vi "Fields filled check.vi"(5 "Module stack name (no hyphens; include 320)":string, 6 "Toplayer ID":string, 7 "Baselayer ID":string) -> (0 "Fields fully (not)filled":bool, 1 "Module stack name (no hyphens; include 320) out":string, 2 "Toplayer ID out":string, 3 "Baselayer ID  out":string)   [LabVIEW 2022 SP3, in "Stack.lvclass"]
uses:
  Stack.lvclass
  <vilib>/Utility/error.llb/Trim Whitespace One-Sided.vi
panel:
  out "All not empty":bool
  out "Both not empty":bool
  out "module not empty":bool
  out "module empty":bool
  out "Both empty":bool
  out "All empty":bool
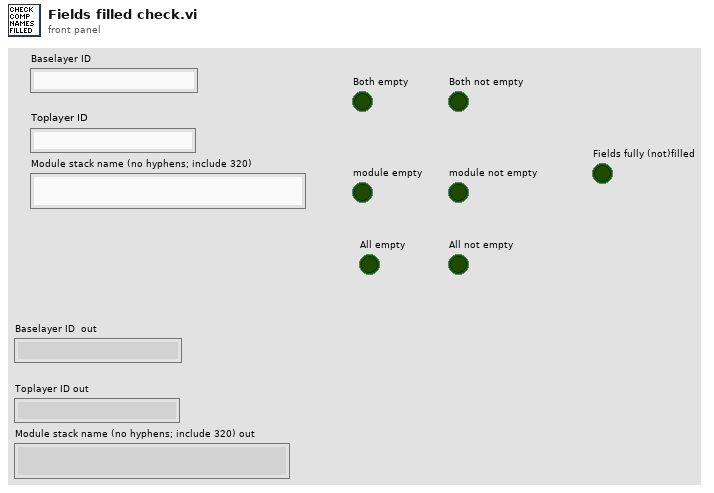
[diagram p1: front panel]
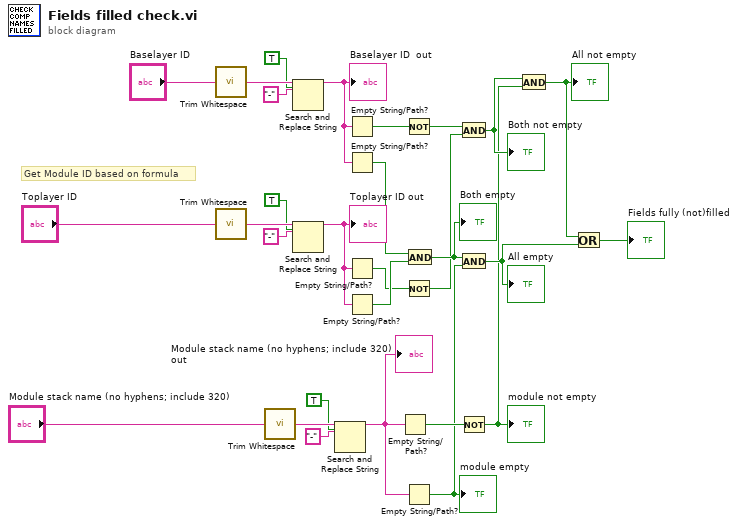
[diagram p0: block diagram]
diagram:
  # "Get Module ID based on formula"
  n1 = call <vilib>:"Trim Whitespace.vi"("string"="Baselayer ID") -> ("trimmed string"=w25:string)  [unwired: 1 in]
  n2 = call <vilib>:"Trim Whitespace.vi"("string"="Toplayer ID") -> ("trimmed string"=w24:string)  [unwired: 1 in]
  n3 = call <vilib>:"Trim Whitespace.vi"("string"="Module stack name (no hyphens; include 320)") -> ("trimmed string"=w27:string)  [unwired: 1 in]
  n4 = Search and Replace String(replace all?=TRUE ("replace all? (F)"), input string=w25, search string="-") -> (result string=w4:string)  [unwired: 5 in, 3 out]
  "Baselayer ID  out" <- w4
  n5 = Search and Replace String(replace all?=TRUE ("ignore case? (F)"), input string=w24, search string="-") -> (result string=w1:string)  [unwired: 5 in, 3 out]
  "Toplayer ID out" <- w1
  n6 = Search and Replace String(replace all?=TRUE ("replace all? (F)"), input string=w27, search string="-") -> (result string=w7:string)  [unwired: 5 in, 3 out]
  "Module stack name (no hyphens; include 320) out" <- w7
  n7 = Empty String/Path?(string/path=w4) -> (empty?=w9:bool)
  n8 = Empty String/Path?(string/path=w4) -> (empty?=w12:bool)
  n9 = Empty String/Path?(string/path=w1) -> (empty?=w10:bool)
  n10 = Empty String/Path?(string/path=w1) -> (empty?=w11:bool)
  n11 = Empty String/Path?(string/path=w7) -> (empty?=w8:bool)
  n12 = Not(x=w9) -> (.not. x?=w3:bool)
  n13 = Not(x=w10) -> (.not. x?=w2:bool)
  n14 = Empty String/Path?(string/path=w7) -> (empty?=w6:bool)
  "module empty" <- w6
  n15 = And(x=w12, y=w11) -> (x .and. y?=w28:bool)
  "Both empty" <- w28
  n16 = And(x=w3, y=w2) -> (x .and. y?=w13:bool)
  "Both not empty" <- w13
  n17 = And(x=w28, y=w6) -> (x .and. y?=w29:bool)
  "All empty" <- w29
  n18 = Not(x=w8) -> (.not. x?=w5:bool)
  "module not empty" <- w5
  n19 = And(x=w13, y=w5) -> (x .and. y?=w14:bool)
  "All not empty" <- w14
  n20 = Or(x=w14, y=w29) -> (x .or. y?=→"Fields fully (not)filled":bool)
